vi "Resolve Timestamp Format__ogtk.vi"(1 "Timestamp Format In":string) -> (0 "Timestamp Format Out":string)   [LabVIEW 2016]
doc: "Resolves a <b>Timestamp Format</b> string. <b>ISO 8601</b> is used as the default formating for Timestamp unless otherwise specified.\n\n<b>ISO 8601</b> is used with the following options: \n Extended format\n UTC\n Decimal point (.) for decimal fractions (lowest order of time element is seconds)\n 3 Decimal places\n<b>E.g:</b> [YYYY]-[MM]-[DD]T[hh]:[mm]:[ss]Z\n\nThis VI is <b>Private</b>."
uses:
  <userlib>/_OpenG.lib/string/string.llb/Trim Whitespace (String)__ogtk.vi
panel:
  # "Please visit http://www.OpenG.org to learn about the\nOpen Source LabVIEW software movement.\n\nNOTICE -- YOU MUST LEAVE THIS NOTICE IN PLACE.  PER THE TERMS OF THE LICENSE BELOW, YOU MAY SUBLICENSE THIS SOFTWARE \nIN ANY WAY THAT DOES NOT CONFLICT WITH THIS LICENSE.\n\n### BSD License (http://www.opensource.org/licenses/bsd-license.php) Begin ###\n \nCopyright (c) 2011, Jonathon Green <jg@jgcode.net>\nCopyright (c) 2011, Phillip Brooks <pbrooks100@gmail.com>\nCopyright (c) 2011, Jonas Mellroth<jonas.mellroth@wireflow.se>\n\nAll rights reserved.\n\nRedistribution and use in source and binary forms, with or without modification, are permitted provided that the following conditions are met:\n\n    * Redistributions of source code must retain the above copyright notice, this list of conditions and the following disclaimer.\n    * Redistributions in binary form must reproduce the above copyright notice, this list of conditions and the following disclaimer in the \n       documentation and/or other materials provided with the distribution.\n    * Neither the name of SciWare, James Kring, Inc., nor the names of its contributors may be used to endorse or promote products derived \n       from this software without specific prior written permission.\n\nTHIS SOFTWARE IS PROVIDED BY THE COPYRIGHT HOLDERS AND CONTRIBUTORS \"AS IS\" AND ANY EXPRESS OR IMPLIED WARRANTIES, \nINCLUDING, BUT NOT LIMITED TO, THE IMPLIED WARRANTIES OF MERCHANTABILITY AND FITNESS FOR A PARTICULAR PURPOSE ARE \nDISCLAIMED. IN NO EVENT SHALL THE COPYRIGHT OWNER OR CONTRIBUTORS BE LIABLE FOR ANY DIRECT, INDIRECT, INCIDENTAL,\n SPECIAL, EXEMPLARY, OR CONSEQUENTIAL DAMAGES (INCLUDING, BUT NOT LIMITED TO, PROCUREMENT OF SUBSTITUTE GOODS OR \nSERVICES; LOSS OF USE, DATA, OR PROFITS; OR BUSINESS INTERRUPTION) HOWEVER CAUSED AND ON ANY THEORY OF LIABILITY, \nWHETHER IN CONTRACT, STRICT LIABILITY, OR TORT (INCLUDING NEGLIGENCE OR OTHERWISE) ARISING IN ANY WAY OUT OF THE USE \nOF THIS SOFTWARE, EVEN IF ADVISED OF THE POSSIBILITY OF SUCH DAMAGE.\n\n### BSD License End ###"
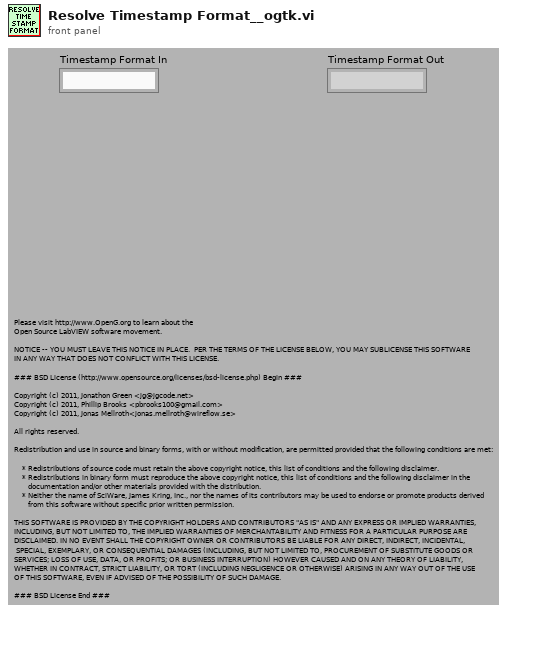
[diagram p1: front panel]
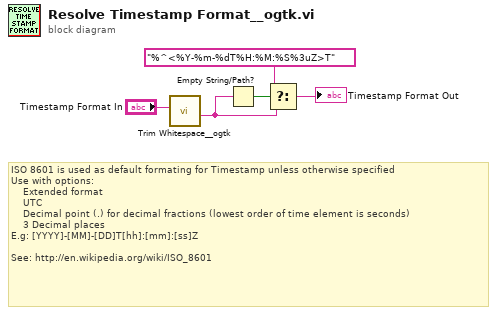
[diagram p0: block diagram]
diagram:
  # "ISO 8601 is used as default formating for Timestamp unless otherwise specified\nUse with options: \n    Extended format\n    UTC\n    Decimal point (.) for decimal fractions (lowest order of time element is seconds)\n    3 Decimal places\nE.g: [YYYY]-[MM]-[DD]T[hh]:[mm]:[ss]Z\n\nSee: http://en.wikipedia.org/wiki/ISO_8601"
  n1 = call-poly <userlib>:"Trim Whitespace__ogtk.vi"("String in"="Timestamp Format In") -> ("String out"=w1:string)  [unwired: 6 in]
  n2 = Empty String/Path?(string/path=w1) -> (empty?=w5:bool)
  n3 = Select(t="%^<%Y-%m-%dT%H:%M:%S%3uZ>T" ("Format String"), s=w5, f=w1) -> (s? t:f=→"Timestamp Format Out":string)
